vi "rs3 get frame data2.vi"(8 "error in (no error)":errorcluster, 9 "size":cluster{"width":u32, "height":u32}, 10 "stream type":u16(ring) items=["depth", "color", "inf 1", "inf 2"], 11 "device in":u64) -> (0 "error out":errorcluster, 1 "2D Color Output":u32[][](array[numeric]), 2 "2D Depth Output":u16[][](array[numeric]), 3 "device out":u64, 5 "image pointer out":u64)   [LabVIEW 2023]
doc: "With a FRAME handle as input, this will return a pointer to the actual image data. \nUse the different MEMCOPY VIs to copy the data into LabVIEW."
panel:
  # "RS3 Get Frame Data 2"
  # "(C) Intel Corp. 2017,  AGJ"
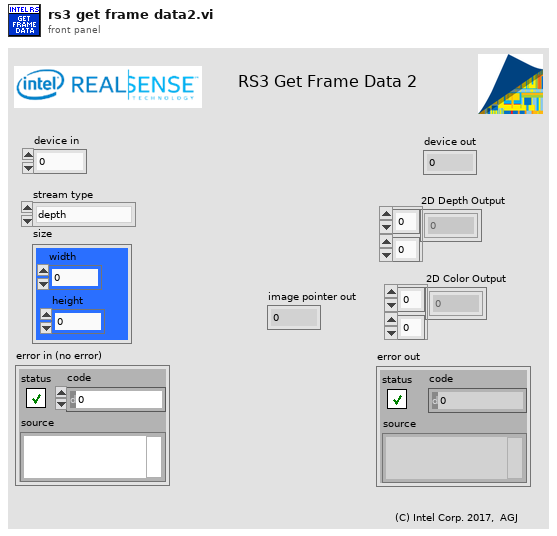
[diagram p1: front panel]
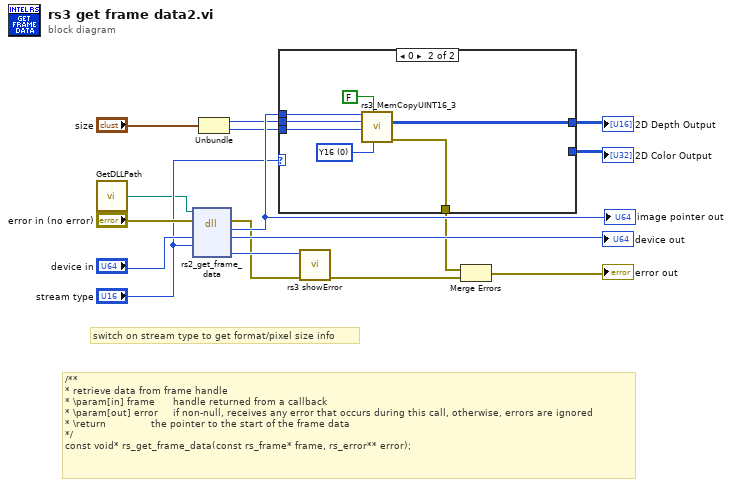
[diagram p0: block diagram]
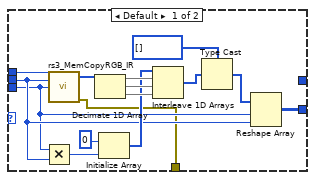
[diagram p2: hidden frame]
diagram:
  # "switch on stream type to get format/pixel size info"
  # "/**\n* retrieve data from frame handle\n* \\param[in] frame      handle returned from a callback\n* \\param[out] error     if non-null, receives any error that occurs during this call, otherwise, errors are ignored\n* \\return               the pointer to the start of the frame data\n*/\nconst void* rs_get_frame_data(const rs_frame* frame, rs_error** error);"
  n1 = call "GetDLLPath.vi"() -> ("DLL Path"=w1:path)
  n2 = dll-call lib="C:/STEAMSyndicate/RealSenseWrappers/VI Wrappers (add ons) Public/RealSense/realsense2.dll" fn="rs2_get_frame_data"(path in=w1, error in="error in (no error)", "device"="device in", "streamType"="stream type") -> (error out=w11:errorcluster, "return type"=w13:u64, "device"=→"device out":u64, "error"=w12:u64)  [unwired: 3 in, 1 out]
  "image pointer out" <- w13
  n3 = Unbundle("size") -> ("width"=w7:u32, "height"=w6:u32)
  n4 = case shown="0" "stream type" {
    tunnel: w13 -> [w31 w38]
    tunnel: [_ w36] -> w9
    tunnel: w7 -> [w22 w34]
    tunnel: w6 -> [w21 w33]
    tunnel: [w25 _] -> w5
    tunnel: [w17 w32] -> w2
    frame Default {
      n5 = Multiply(x=w21, y=w22) -> (x*y=w24:u32)
      n6 = call "rs3_MemCopyRGB_IR.vi"("Zimage pointer"=w31, "RGB  X, width"=w22, "RGB Y, height"=w21) -> ("Output Array"=w30:u8[], "error out"=w17:errorcluster)  [unwired: 11 in]
      n7 = Decimate 1D Array(w30) -> (w29:u8[], w28:u8[], w27:u8[])
      n8 = Initialize Array(u8 0, w24) -> (w23:u8[])
      n9 = Interleave 1D Arrays(w23, w29, w28, w27) -> (w20:u8[])
      n10 = Type Cast(type=u32[] [], x=w20) -> (*(type *) &x=w19:u32[])
      n11 = Reshape Array(w19, w21, w22) -> (w25:u32[][])
    }
    frame 0 {
      w37 = u16 0 items=["Y16", "Y8"] ("Image format")
      n12 = call "rs3_MemCopyUINT16_3.vi"("Image format"=w37, "Transpose"=FALSE, "Height"=w33, "Width"=w34, "Zimage pointer"=w38) -> ("error out"=w32:errorcluster, "2D Array Output"=w36:u16[][])  [unwired: 5 in]
    }
  }
  "2D Depth Output" <- w9
  "2D Color Output" <- w5
  n13 = call "rs3 showError.vi"("error in (no error)"=w11, "error"=w12) -> ("error out"=w3:errorcluster)  [unwired: 5 in, 4 out]
  n14 = Merge Errors(w2, w3) -> (→"error out":errorcluster)
